vi "MIMIC Port Init.vi"(2 "MIMIC TIMEOUT":u32, 3 "MIMC BAUD":u32=9600, 4 "MIMIC_PORT":refnum<visa-resource-name>="COM1") -> (0 "error out":errorcluster, 1 "MIMIC PORT RESOURCE":refnum<visa-resource-name>)   [LabVIEW 2014]
uses:
  <vilib>/Instr/_visa.llb/VISA Flush IO Buffer Mask.ctl
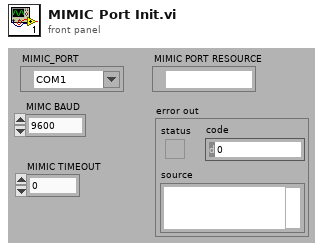
[diagram p1: front panel]
types:
  T1 = enum16{"Initial Serial Port", "Write", "Read", "Close", "ClearBuff"}
  T2 = typedef "VISA Flush IO Buffer Mask.ctl" = u16
  T3 = cluster{"MIMIC TIMEOUT":u32, "MIMC BAUD":u32, "data bits":u16, "parity (0:none)":enum16{"None", "Odd", "Even", "Mark", "Space"}, "stop bits (10: 1 bit)":u16}
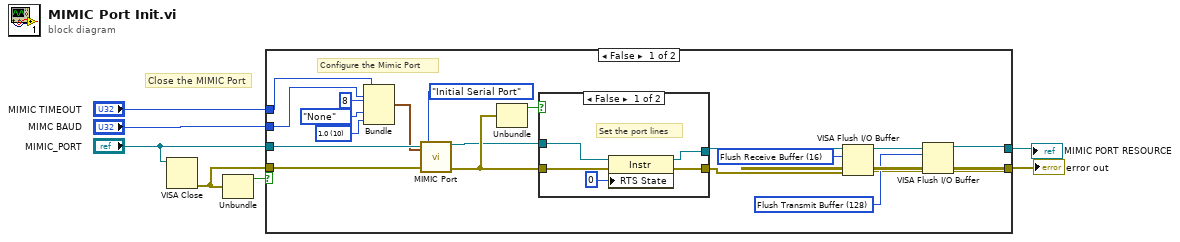
[diagram p0: block diagram]
diagram:
  # "Close the MIMIC Port"
  n1 = VISA Close ("Close MIMIC Port")(VISA resource name="MIMIC_PORT") -> (error out=w7:errorcluster)  [unwired: 1 in]
  n2 = Unbundle(w7) -> ("status"=w6:bool)  [unwired: 2 out]
  n3 = case shown="False" w6 {
    tunnel: [w11 w34] -> w2
    tunnel: w7 -> [w26 w34]
    tunnel: "MIMIC_PORT" -> [w24 _]
    tunnel: "MIMC BAUD" -> [w23 _]
    tunnel: "MIMIC TIMEOUT" -> [w17 _]
    tunnel: [w12 _] -> w1
    frame False {
      w9 = T2 128 items=["Flush Receive Buffer"=16, "Write Transmit Buffer to Device"=32, "Flush Receive Buffer (No I/O)"=64, "Flush Transmit Buffer"=128] ("Mask")
      w13 = T2 16 items=["Flush Receive Buffer"=16, "Write Transmit Buffer to Device"=32, "Flush Receive Buffer (No I/O)"=64, "Flush Transmit Buffer"=128] ("Mask")
      w20 = u16 10 items=["1.0"=10, "1.5"=15, "2.0"=20] ("stop bits (10: 1 bit)")
      # "Configure the Mimic Port"
      n4 = Bundle("MIMIC TIMEOUT"=w17, "MIMC BAUD"=w23, "data bits"=u16 8, "parity (0:none)"=enum16{"None", "Odd", "Even", "Mark", "Space"}."None", "stop bits (10: 1 bit)"=w20) -> (w19:T3)  [unwired: 1 in]
      n5 = call "MIMIC Port.vi"("VISA resource name"=w24, "Port Setting"=w19, "error in (no error)"=w26, "Function"=T1."Initial Serial Port") -> ("output VISA resource name"=w16:refnum<visa-resource-name>, "error out"=w25:errorcluster)  [unwired: 12 in, 2 out]
      n6 = Unbundle(w25) -> ("status"=w27:bool)  [unwired: 2 out]
      n7 = case shown="False" w27 {
        tunnel: w25 -> [w29 w33]
        tunnel: [w30 w33] -> w14
        tunnel: w16 -> [w32 _]
        tunnel: [w28 _] -> w15
        frame False {
          # "Set the port lines"
          n8 = property class="Instr"(reference=w32, error in=w29, "RTS State"=i16 0) -> (reference out=w28:refnum<visa-resource-name>, error out=w30:errorcluster)
        }
        frame True {
        }
      }
      n9 = VISA Flush I/O Buffer(VISA resource name=w15, mask (16)=w13, error in (no error)=w14) -> (VISA resource name out=w10:refnum<visa-resource-name>, error out=w8:errorcluster)
      n10 = VISA Flush I/O Buffer(VISA resource name=w10, mask (16)=w9, error in (no error)=w8) -> (VISA resource name out=w12:refnum<visa-resource-name>, error out=w11:errorcluster)
    }
    frame True {
    }
  }
  "error out" <- w2
  "MIMIC PORT RESOURCE" <- w1
